vi "Message Queue Status.vi"(8 "error in (no error)":errorcluster, 11 "Message Queue":refnum<queue>) -> (0 "error out":errorcluster, 3 "dup Message Queue":refnum<queue>)   [LabVIEW 2014, in "UI_ProgressDlg.lvlib" / "UI_ProgressDlg.lvclass"]
doc: "This VI pulls messages off the Message Queue. It has special error handling to account for an error occurring on the last iteration of the Message Handling Loop.\n\nNo Error - normal Dequeue Element operation.\nError - check if it is an error code we wish to ignore. If so, clear the error and perform a normal Dequeue Element. If not, output the error, and put a 'Stop' message on the Message Queue."
uses:
  UI_ProgressDlg.lvclass
  Message Cluster.ctl
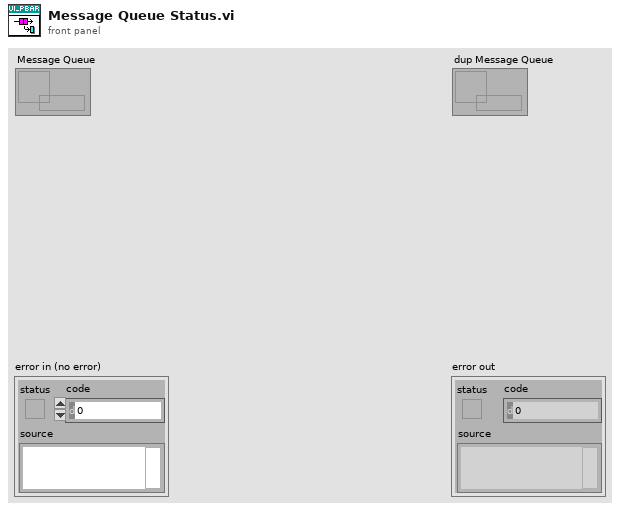
[diagram p1: front panel]
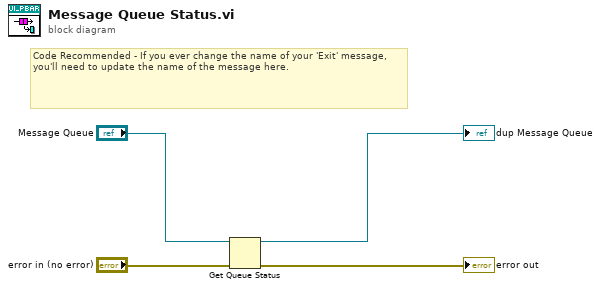
[diagram p0: block diagram]
diagram:
  # "Code Recommended - If you ever change the name of your 'Exit' message, you'll need to update the name of the message here."
  n1 = Get Queue Status(queue="Message Queue", error in (no error)="error in (no error)") -> (queue out=→"dup Message Queue":refnum<queue>, error out=→"error out":errorcluster)  [unwired: 1 in, 6 out]
